vi "GetElement(Single).vi"(7 "Qualified Name":string, 8 "error in (no error)":errorcluster, 10 "Key":string, 11 "ConfigManager.Cache in":refnum<class "ConfigManager.Cache.lvclass">) -> (0 "error out":errorcluster, 1 "found":bool, 2 "Value":string, 3 "ConfigManager.Cache out":refnum<class "ConfigManager.Cache.lvclass">)   [LabVIEW 2013, in "CfgManager.lvlib" / "ConfigManager.Cache.lvclass"]
uses:
  ConfigManager.Cache.lvclass
  ConfigManager.Cache.lvclass/ConfigManager.Cache.ctl
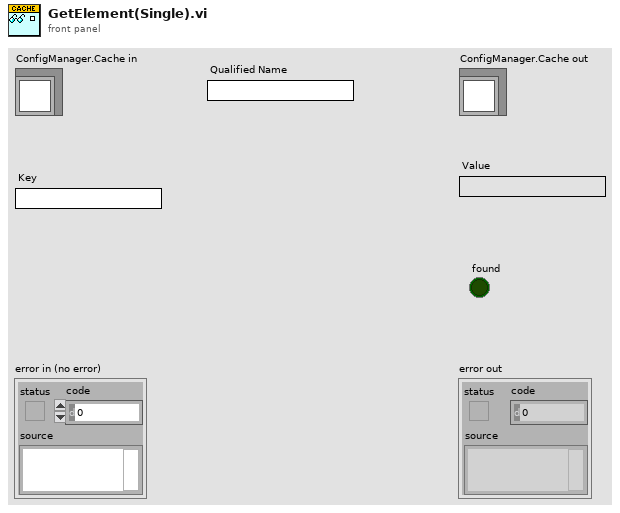
[diagram p1: front panel]
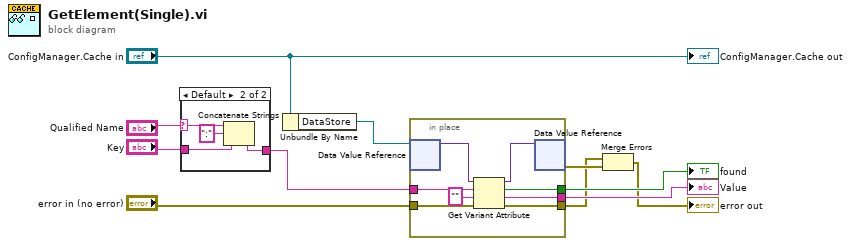
[diagram p0: block diagram]
diagram:
  n1 = case shown="Default" "Qualified Name" {
    selector: "Qualified Name" -> [_ w13]
    tunnel: "Key" -> [w12 w15]
    tunnel: [w12 w14] -> w7
    frame "" {
    }
    frame Default {
      n2 = Concatenate Strings(w13, ":" ("string"), w15) -> (w14:string)
    }
  }
  n3 = Unbundle By Name("ConfigManager.Cache in") -> ("DataStore"=w1:refnum<data-value>)
  n4 = in-place {
    in-place-border: "error in (no error)" -> [w24]
    in-place-border: w7 -> [w23]
    in-place-border: [w22] -> w3
    in-place-border: [w20] -> w10
    in-place-border: [w19] -> w9
    n5 = in-place-dvr #1(w1) -> (w18:variant)  [unwired: 1 out]
    n6 = Get Variant Attribute(Variant=w18, name=w23, default value (empty Variant)="", error in=w24) -> (duplicate Variant=w17:variant, found=w19:bool, value=w20:string, error out=w22:errorcluster)
    n7 = in-place-dvr #1(w17) -> (w5:errorcluster)  [unwired: 1 out]
  }
  "Value" <- w10
  "found" <- w9
  n8 = Merge Errors(w3, w5) -> (→"error out":errorcluster)
  "ConfigManager.Cache out" <- "ConfigManager.Cache in"
